vi "Remove Channel.vi"(8 "error in (no error)":errorcluster, 10 "ID":string, 11 "Configuration Session in":refnum<class "Configuration.lvclass">) -> (0 "error out":errorcluster, 3 "Configuration Session out":refnum<class "Configuration.lvclass">, 4 "exists?":bool)   [LabVIEW 2017, in "DSF Core.lvlib" / "Configuration.lvclass"]
doc: "Removes a section from the configuration data identified by <B>dsf refnum</B>."
uses:
  Configuration.lvclass
  Configuration.lvclass/Configuration.ctl
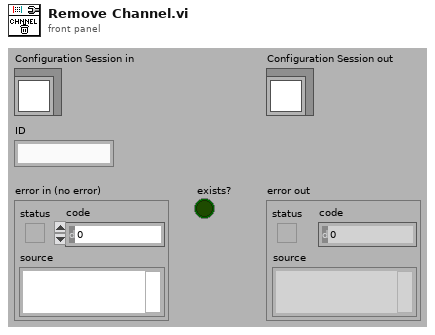
[diagram p1: front panel]
types:
  T1 = typedef "DSF Core.lvlib/Configuration.lvclass/DSF Config Data Ref.ctl" = refnum<data-value>
  T2 = typedef "DSF Core.lvlib/Configuration.lvclass/DSF Config Data.ctl" = cluster{"dsf configuration":T3, "path":path, "dirty":bool}
  T3 = typedef "DSF Core.lvlib/Configuration.lvclass/Internal DSF Configuration.ctl" = cluster{"dsfversion":T4, "version":T4, "plugins":T5[], "groups":T10[], "transfers":T12[], "channels":T14[], "settings":T16[]}
  T4 = typedef "DSF Core.lvlib/DSF Version Info.ctl" = cluster{"major":u32, "minor":u32, "fix":u32, "build":string}
  T5 = typedef "DSF Core.lvlib/Configuration.lvclass/Internal DSF Plugin with ID.ctl" = cluster{"id":string, "values":T6}
  T6 = typedef "DSF Core.lvlib/Configuration.lvclass/Internal DSF Plugin Info.ctl" = cluster{"components":string[], "timing":T7, "group ids":string[], "settings id":string, "threads":T8[]}
  T7 = typedef "DSF Core.lvlib/DSF Timing Info.ctl" = cluster{"priority":u64, "decimation":u64, "offset":u64}
  T8 = typedef "DSF Core.lvlib/DSF Engine Plugin Thread Configuration.ctl" = cluster{"buffer converter settings":T9, "transceiver settings":T9, "processor":i32, "priority offset":i16}
  T9 = typedef "DSF Core.lvlib/DSF Settings Info.ctl" = cluster{"key":string, "value":string}[]
  T10 = typedef "DSF Core.lvlib/Configuration.lvclass/Internal DSF Group with ID.ctl" = cluster{"id":string, "values":T11}
  T11 = typedef "DSF Core.lvlib/Configuration.lvclass/Internal DSF Group Info.ctl" = cluster{"direction":i32, "timing":T7, "transfer ids":string[], "settings id":string, "thread":i32, "timeout behavior":u8}
  T12 = typedef "DSF Core.lvlib/Configuration.lvclass/Internal DSF Transfer with ID.ctl" = cluster{"id":string, "values":T13}
  T13 = typedef "DSF Core.lvlib/Configuration.lvclass/Internal DSF Transfer Info.ctl" = cluster{"byte order":i32, "channel ids":string[], "settings id":string}
  T14 = typedef "DSF Core.lvlib/Configuration.lvclass/Internal DSF Channel with ID.ctl" = cluster{"id":string, "values":T15}
  T15 = typedef "DSF Core.lvlib/Configuration.lvclass/Internal DSF Channel Info.ctl" = cluster{"string buffer offset":u64, "string data type":i32, "engine data type":i32, "settings id":string}
  T16 = typedef "DSF Core.lvlib/Configuration.lvclass/Internal DSF Settings with ID.ctl" = cluster{"id":string, "values":T17}
  T17 = typedef "DSF Core.lvlib/Configuration.lvclass/Internal DSF Settings Info.ctl" = cluster{"key":string, "value":string}[]
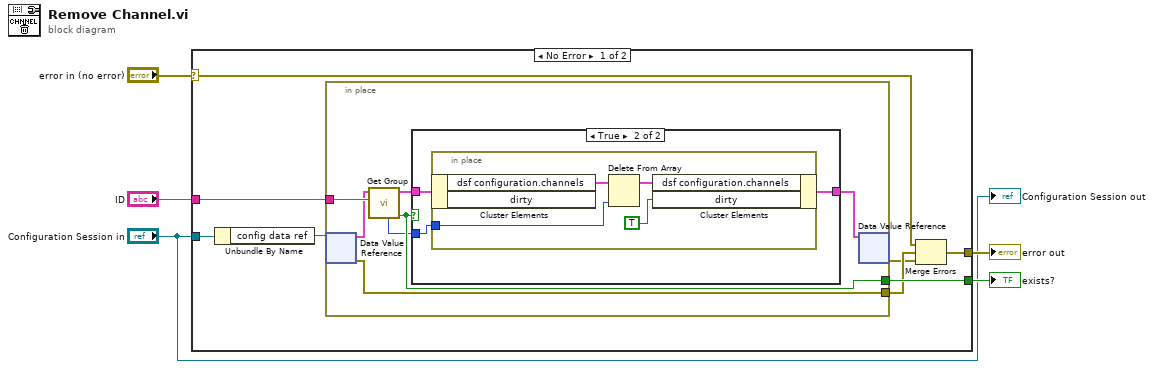
[diagram p0: block diagram]
diagram:
  n1 = case shown="No Error" "error in (no error)" {
    selector: "error in (no error)" -> [w11 w29]
    tunnel: [w10 w29] -> w2
    tunnel: "Configuration Session in" -> [w7 _]
    tunnel: "ID" -> [w13 _]
    tunnel: [w12 _] -> w3
    frame No Error {
      n2 = Unbundle By Name(w7) -> ("config data ref"=w6:T1)
      n3 = in-place {
        in-place-border: w13 -> [w20]
        in-place-border: [w19] -> w12
        in-place-border: [w14] -> w9
        n4 = in-place-dvr #1(w6) -> (w16:T2, w14:errorcluster)
        n5 = call "Get Group.vi"("id"=w20, "DSF Configuration in"=w16) -> ("exists?"=w19:bool, "DSF Configuration out"=w18:T2, "index"=w17:i32)  [unwired: 6 in, 1 out]
        n6 = case shown="True" w19 {
          tunnel: [w21 w24] -> w15
          tunnel: w17 -> [_ w23]
          tunnel: w18 -> [w21 w22]
          frame False {
          }
          frame True {
            n7 = in-place {
              in-place-border: w23 -> [w28]
              n8 = in-place-cluster #2(w22) -> ("dsf configuration.channels"=w27:T14[])  [unwired: 1 out]
              n9 = Delete From Array(array=w27, index=w28) -> (array with subset deleted=w26:T14[])  [unwired: 1 in, 1 out]
              n10 = in-place-cluster #2("dsf configuration.channels"=w26, "dirty"=TRUE) -> (w24:T2)
            }
          }
        }
        n11 = in-place-dvr #1(w15) -> (w8:errorcluster)  [unwired: 1 out]
      }
      n12 = Merge Errors(w11, w9, w8) -> (w10:errorcluster)
    }
    frame Error {
    }
  }
  "error out" <- w2
  "exists?" <- w3
  "Configuration Session out" <- "Configuration Session in"
